vi "path2string.vi"(11 "folder path":path) -> (3 "String":string)   [LabVIEW 2017]
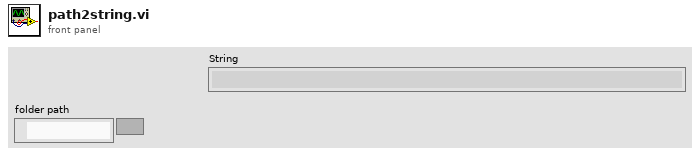
[diagram p1: front panel]
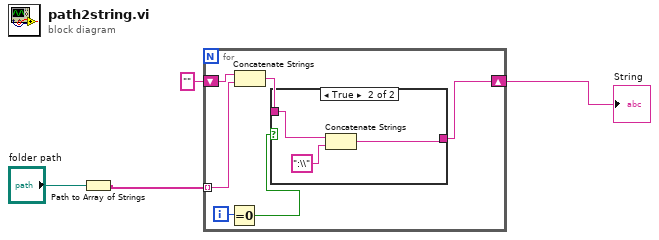
[diagram p0: block diagram]
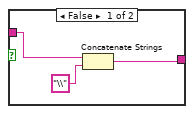
[diagram p2: hidden frame]
diagram:
  n1 = Path to Array of Strings(0:"folder path") -> (2:w1:string[])  [unwired: 1 out]
  n2 = for {
    tunnel: w1 -> [w6] mode=indexing
    shift-right: [w8] -> w3
    shift-left: "" -> [w7]
    i -> [w9]
    n3 = Equal To 0?(x=w9) -> (x = 0?=w10:bool)
    n4 = Concatenate Strings(w7, w6) -> (w5:string)
    n5 = case shown="True" w10 {
      tunnel: [w12 w15] -> w8
      tunnel: w5 -> [w11 w14]
      frame False {
        n6 = Concatenate Strings(w11, "\\" ("string")) -> (w12:string)
      }
      frame True {
        n7 = Concatenate Strings(w14, ":\\" ("string")) -> (w15:string)
      }
    }
  }
  "String" <- w3
